vi "PicoReadPicoMultiBuffers.vi"(1 "enabled array":i16[](array[numeric]), 2 "Buffer and Transfer Settings":T3={"startIndex"=0, "Samples"=1000000, "Down Sample Ratio"=1, "Down-Sample Mode"=2147483648} {"Down-Sample Mode" items=["RAW none"=2147483648, "None"=0, "Aggregate"=1, "Decimate"=2, "Average"=4]; "Down Sample Ratio" step=1; "Samples" format="%_6p"}, 3 "Variant":string, 5 "Data Pointers":T1, 9 "No of Buffers":i32=1, 11 "error in (no error)":errorcluster) -> (6 "MultiBuffers (Max or non-aggregated)":T2(array[cluster]), 8 "Min Buffers":T2(array[cluster]), 15 "error out":errorcluster)   [LabVIEW 2024]
doc: "Read data from Picodata buffers for Block and 6000a streaming examples"
uses:
  Buffer and Transfer Settings.ctl
  PicoBuffers.ctl
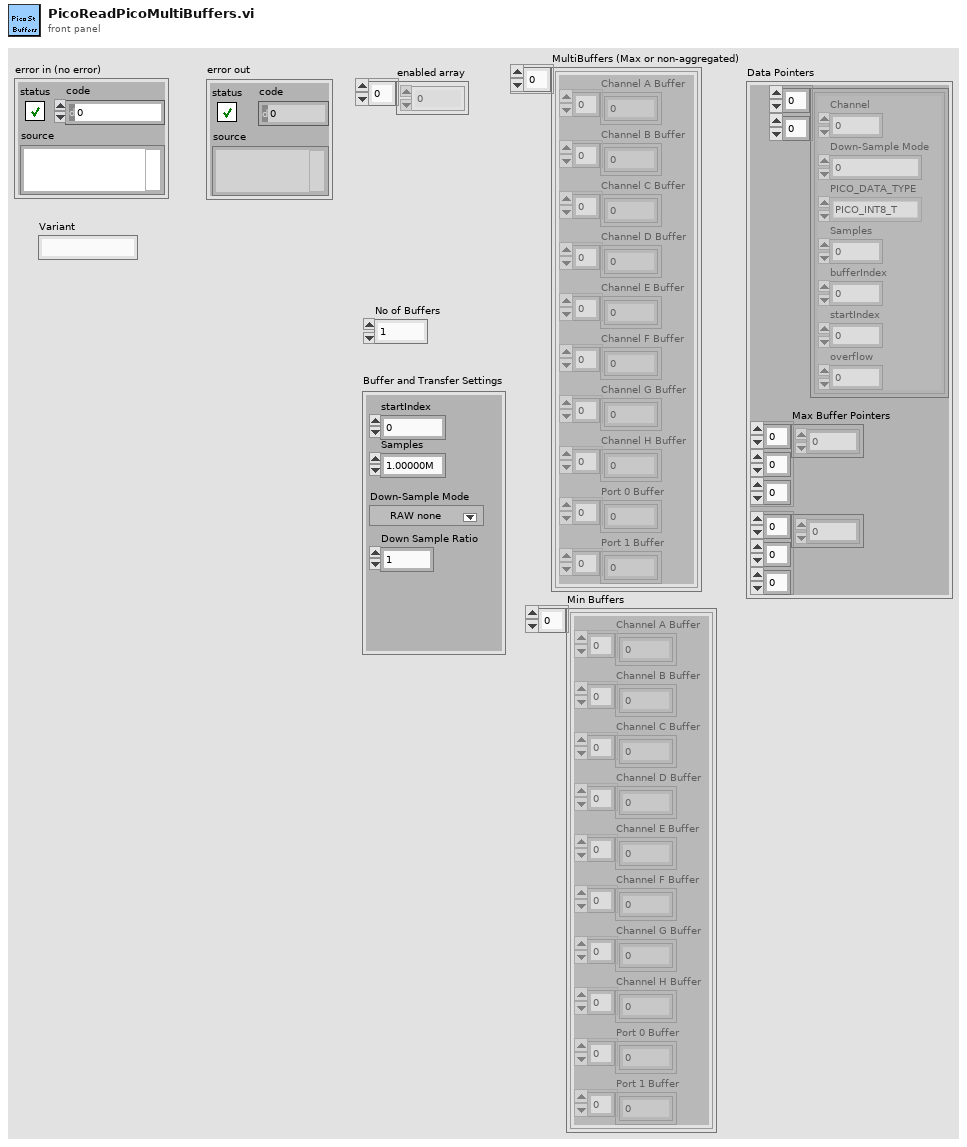
[diagram p1: front panel]
types:
  T1 = typedef "PicoBuffers.ctl" = cluster{"Max Buffer Pointers":u64[][][], "Min Buffer Pointers":u64[][][], "StreamingDataInfo":cluster{"Channel":u32, "Down-Sample Mode":u32, "PICO_DATA_TYPE":enum32{"PICO_INT8_T", "PICO_INT16_T", "PICO_INT32_T", "PICO_UINT32_T", "PICO_INT64_T", ""}, "Samples":i32, "bufferIndex":u64, "startIndex":i32, "overflow":i16}[][]}
  T2 = cluster{"Channel A Buffer":i16[], "Channel B Buffer":i16[], "Channel C Buffer":i16[], "Channel D Buffer":i16[], "Channel E Buffer":i16[], "Channel F Buffer":i16[], "Channel G Buffer":i16[], "Channel H Buffer":i16[], "Port 0 Buffer":i16[], "Port 1 Buffer":i16[]}[]
  T3 = typedef "Buffer and Transfer Settings.ctl" = cluster{"startIndex":u64, "Samples":u64, "Down Sample Ratio":u64, "Down-Sample Mode":u32}
  T4 = cluster{"Channel A Buffer":i16[], "Channel B Buffer":i16[], "Channel C Buffer":i16[], "Channel D Buffer":i16[], "Channel E Buffer":i16[], "Channel F Buffer":i16[], "Channel G Buffer":i16[], "Channel H Buffer":i16[], "Port 0 Buffer":i16[], "Port 1 Buffer":i16[]}
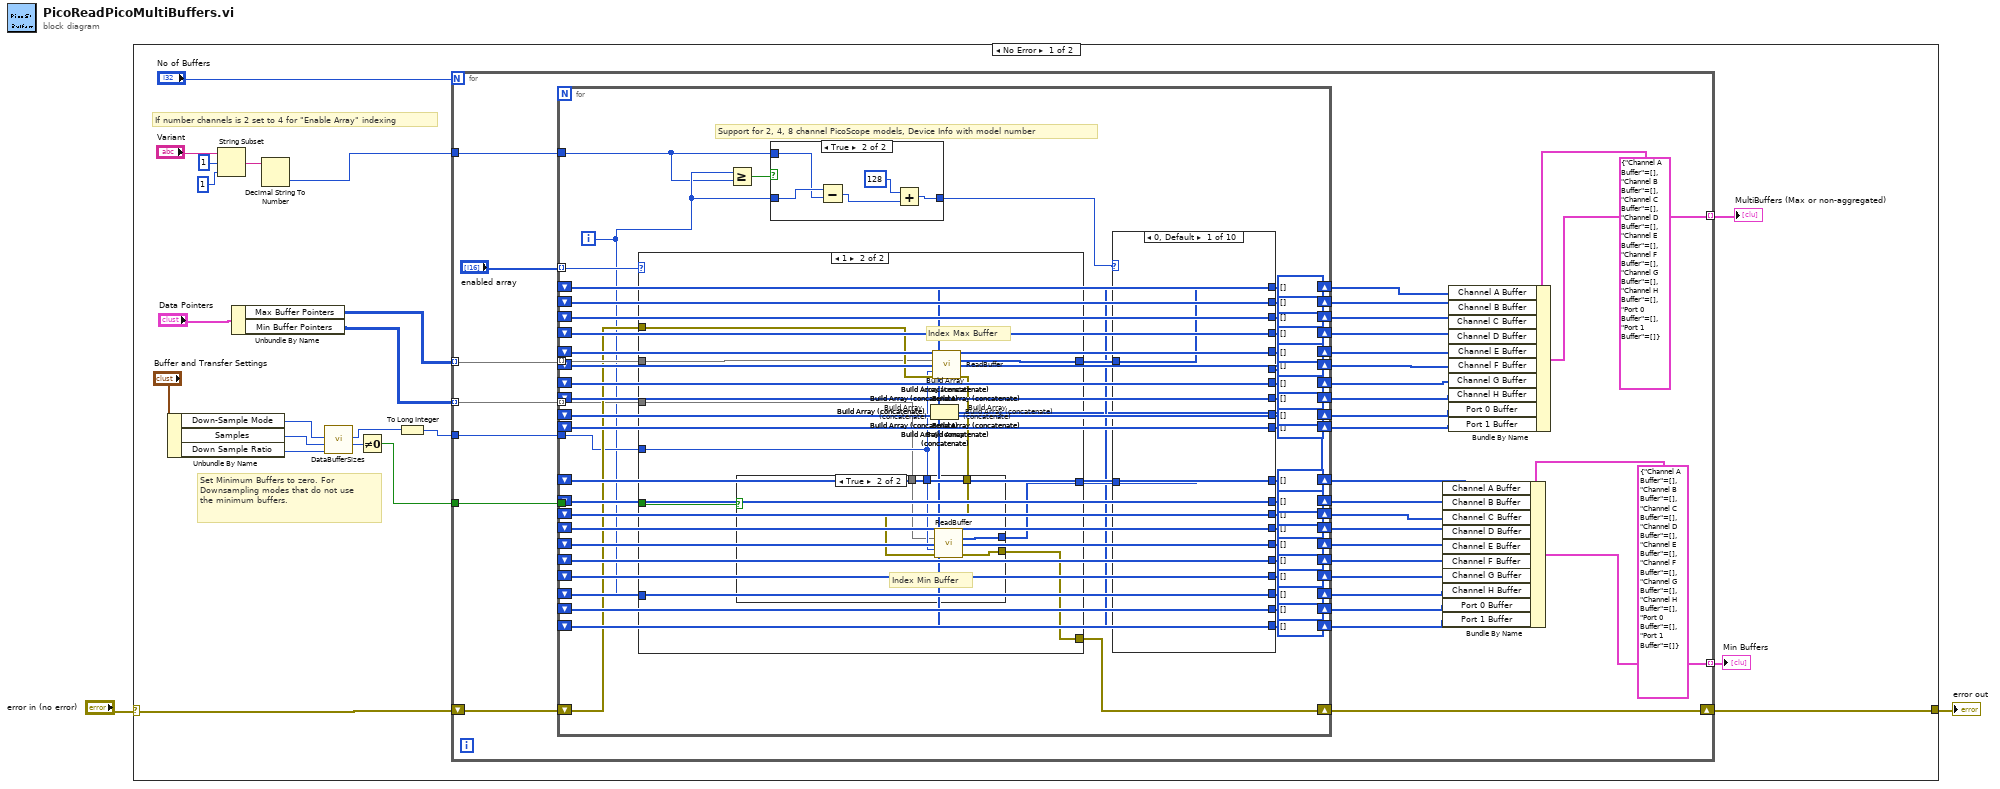
[diagram p0: block diagram]
diagram:
  n1 = case shown="No Error" "error in (no error)" {
    selector: "error in (no error)" -> [w21 w191]
    tunnel: [w23 w191] -> w1
    frame No Error {
      # "If number channels is 2 set to 4 for \"Enable Array\" indexing"
      # "Set Minimum Buffers to zero. For Downsampling modes that do not use the minimum buffers."
      n2 = Unbundle By Name("Buffer and Transfer Settings") -> ("Down-Sample Mode"=w19:u32, "Samples"=w18:u64, "Down Sample Ratio"=w20:u64)
      n3 = String Subset(string="Variant", offset (0)=1, length (rest)=1 ("length (rest)")) -> (substring=w7:string)
      n4 = Unbundle By Name("Data Pointers") -> ("Max Buffer Pointers"=w9:u64[][][], "Min Buffer Pointers"=w8:u64[][][])
      n5 = Decimal String To Number(string=w7) -> (number=w3:i32)  [unwired: 2 in, 1 out]
      n6 = call "DataBufferSizes.vi"("Down Sample Ratio"=w20, "Number of Samples"=w18, "Down-Sample Mode"=w19) -> ("min Buffer Size"=w16:i32, "Max Buffer Size"=w12:i32)  [unwired: 7 in]
      n7 = Not Equal To 0?(x=w16) -> (x != 0?=w17:bool)
      n8 = To Long Integer(number=w12) -> (32bit integer=w15:i32)
      n9 = for {
        N: "No of Buffers" -> [_]
        tunnel: [w73] -> w11 mode=indexing
        tunnel: [w72] -> w13 mode=indexing
        tunnel: w17 -> [w60]
        tunnel: w15 -> [w58]
        shift-right: [w75] -> w23
        shift-left: w21 -> [w74]
        tunnel: w9 -> [w57] mode=indexing
        tunnel: w8 -> [w46] mode=indexing
        tunnel: w3 -> [w45]
        n10 = for {
          tunnel: "enabled array" -> [w147] mode=indexing
          tunnel: w57 -> [w148] mode=indexing
          shift-right: [w146] -> w75
          shift-left: w74 -> [w145]
          tunnel: w58 -> [w131]
          tunnel: w60 -> [w130]
          tunnel: w46 -> [w120] mode=indexing
          tunnel: w45 -> [w116]
          shift-right: [w114] -> w71
          shift-left: i16[] [] ("Output Array") -> [w115]
          shift-right: [w112] -> w70
          shift-left: i16[] [] ("Output Array") -> [w113]
          shift-right: [w110] -> w69
          shift-left: i16[] [] ("Output Array") -> [w111]
          shift-right: [w108] -> w68
          shift-left: i16[] [] ("Output Array") -> [w109]
          shift-right: [w106] -> w67
          shift-left: i16[] [] ("Output Array") -> [w107]
          shift-right: [w104] -> w66
          shift-left: i16[] [] ("Output Array") -> [w105]
          shift-right: [w102] -> w59
          shift-left: i16[] [] ("Output Array") -> [w103]
          shift-right: [w100] -> w65
          shift-left: i16[] [] ("Output Array") -> [w101]
          shift-right: [w98] -> w64
          shift-left: i16[] [] ("Output Array") -> [w99]
          shift-right: [w96] -> w63
          shift-left: i16[] [] ("Output Array") -> [w97]
          shift-right: [w94] -> w62
          shift-left: i16[] [] ("Output Array") -> [w95]
          shift-right: [w92] -> w61
          shift-left: i16[] [] ("Output Array") -> [w93]
          shift-right: [w90] -> w54
          shift-left: i16[] [] ("Output Array") -> [w91]
          shift-right: [w88] -> w53
          shift-left: i16[] [] ("Output Array") -> [w89]
          shift-right: [w86] -> w52
          shift-left: i16[] [] ("Output Array") -> [w87]
          shift-right: [w84] -> w51
          shift-left: i16[] [] ("Output Array") -> [w85]
          shift-right: [w82] -> w50
          shift-left: i16[] [] ("Output Array") -> [w83]
          shift-right: [w80] -> w49
          shift-left: i16[] [] ("Output Array") -> [w81]
          shift-right: [w78] -> w48
          shift-left: i16[] [] ("Output Array") -> [w79]
          shift-right: [w76] -> w47
          shift-left: i16[] [] ("Output Array") -> [w77]
          i -> [w117]
          # "Support for 2, 4, 8 channel PicoScope models, Device Info with model number"
          n11 = case shown="1" w147 {
            tunnel: w148 -> [_ w177]
            tunnel: w117 -> [_ _]
            tunnel: [_ w184] -> w144
            tunnel: [_ w183] -> w143
            tunnel: w145 -> [w175 w182]
            tunnel: [w175 w180] -> w146
            tunnel: w131 -> [_ w178]
            tunnel: w130 -> [_ w179]
            tunnel: w120 -> [_ w176]
            frame 0, Default {
            }
            frame 1 {
              # "Index Max Buffer"
              n12 = call "ReadBuffer.vi"("Pointer and BufferSize"=w177, "Buffer size"=w178, "error in (no error)"=w182) -> ("Output Array"=w184:i16[], "error out"=w181:errorcluster)  [unwired: 11 in]
              n13 = case shown="True" w179 {
                tunnel: [_ w190] -> w183
                tunnel: w181 -> [w185 w189]
                tunnel: [w185 w188] -> w180
                tunnel: w178 -> [_ w187]
                tunnel: w176 -> [_ w186]
                frame False {
                }
                frame True {
                  # "Index Min Buffer"
                  n14 = call "ReadBuffer.vi"("Pointer and BufferSize"=w186, "Buffer size"=w187, "error in (no error)"=w189) -> ("Output Array"=w190:i16[], "error out"=w188:errorcluster)  [unwired: 11 in]
                }
              }
            }
          }
          n15 = Greater Or Equal?(x=w117, y=w116) -> (x >= y?=w119:bool)
          n16 = case shown="True" w119 {
            tunnel: w117 -> [w149 w151]
            tunnel: [w149 w153] -> w118
            tunnel: w116 -> [_ w150]
            frame False {
            }
            frame True {
              n17 = Subtract(x=w151, y=w150) -> (x-y=w152:i32)
              n18 = Add(x=128, y=w152) -> (x+y=w153:i32)
            }
          }
          n19 = case shown="0, Default" w118 {
            tunnel: w144 -> [w156 w158 w160 w162 w164 w166 w168 w170 w172 w174]
            tunnel: [w156 _ _ _ _ _ _ _ _ _] -> w129
            tunnel: [_ w158 _ _ _ _ _ _ _ _] -> w136
            tunnel: [_ _ w160 _ _ _ _ _ _ _] -> w135
            tunnel: [_ _ _ w162 _ _ _ _ _ _] -> w134
            tunnel: [_ _ _ _ w164 _ _ _ _ _] -> w133
            tunnel: [_ _ _ _ _ w166 _ _ _ _] -> w132
            tunnel: w143 -> [w155 w157 w159 w161 w163 w165 w167 w169 w171 w173]
            tunnel: [w155 _ _ _ _ _ _ _ _ _] -> w142
            tunnel: [_ w157 _ _ _ _ _ _ _ _] -> w141
            tunnel: [_ _ w159 _ _ _ _ _ _ _] -> w140
            tunnel: [_ _ _ w161 _ _ _ _ _ _] -> w139
            tunnel: [_ _ _ _ w163 _ _ _ _ _] -> w138
            tunnel: [_ _ _ _ _ w165 _ _ _ _] -> w137
            tunnel: [_ _ _ _ _ _ w168 _ _ _] -> w128
            tunnel: [_ _ _ _ _ _ w167 _ _ _] -> w127
            tunnel: [_ _ _ _ _ _ _ w170 _ _] -> w126
            tunnel: [_ _ _ _ _ _ _ w169 _ _] -> w125
            tunnel: [_ _ _ _ _ _ _ _ w172 _] -> w124
            tunnel: [_ _ _ _ _ _ _ _ w171 _] -> w123
            tunnel: [_ _ _ _ _ _ _ _ _ w174] -> w122
            tunnel: [_ _ _ _ _ _ _ _ _ w173] -> w121
            frame 0, Default {
            }
            frame 1 {
            }
            frame 2 {
            }
            frame 3 {
            }
            frame 4 {
            }
            frame 5 {
            }
            frame 6 {
            }
            frame 7 {
            }
            frame 128 {
            }
            frame 129 {
            }
          }
          n20 = Build Array (concatenate)(w77, w121) -> (w76:i16[])
          n21 = Build Array (concatenate)(w79, w122) -> (w78:i16[])
          n22 = Build Array (concatenate)(w81, w123) -> (w80:i16[])
          n23 = Build Array (concatenate)(w83, w124) -> (w82:i16[])
          n24 = Build Array (concatenate)(w85, w125) -> (w84:i16[])
          n25 = Build Array (concatenate)(w87, w126) -> (w86:i16[])
          n26 = Build Array (concatenate)(w89, w127) -> (w88:i16[])
          n27 = Build Array (concatenate)(w91, w128) -> (w90:i16[])
          n28 = Build Array (concatenate)(w93, w132) -> (w92:i16[])
          n29 = Build Array (concatenate)(w95, w133) -> (w94:i16[])
          n30 = Build Array (concatenate)(w97, w134) -> (w96:i16[])
          n31 = Build Array (concatenate)(w99, w135) -> (w98:i16[])
          n32 = Build Array (concatenate)(w101, w136) -> (w100:i16[])
          n33 = Build Array (concatenate)(w103, w129) -> (w102:i16[])
          n34 = Build Array (concatenate)(w105, w137) -> (w104:i16[])
          n35 = Build Array (concatenate)(w107, w138) -> (w106:i16[])
          n36 = Build Array (concatenate)(w109, w139) -> (w108:i16[])
          n37 = Build Array (concatenate)(w111, w140) -> (w110:i16[])
          n38 = Build Array (concatenate)(w113, w141) -> (w112:i16[])
          n39 = Build Array (concatenate)(w115, w142) -> (w114:i16[])
        }
        n40 = Bundle By Name(cluster=T4 {"Channel A Buffer"=[], "Channel B Buffer"=[], "Channel C Buffer"=[], "Channel D Buffer"=[], "Channel E Buffer"=[], "Channel F Buffer"=[], "Channel G Buffer"=[], "Channel H Buffer"=[], "Port 0 Buffer"=[], "Port 1 Buffer"=[]} ("input cluster"), "Channel A Buffer"=w71, "Channel B Buffer"=w70, "Channel C Buffer"=w69, "Channel D Buffer"=w68, "Channel E Buffer"=w67, "Channel F Buffer"=w66, "Channel G Buffer"=w53, "Channel H Buffer"=w51, "Port 0 Buffer"=w49, "Port 1 Buffer"=w47) -> (w73:T4)
        n41 = Bundle By Name(cluster=T4 {"Channel A Buffer"=[], "Channel B Buffer"=[], "Channel C Buffer"=[], "Channel D Buffer"=[], "Channel E Buffer"=[], "Channel F Buffer"=[], "Channel G Buffer"=[], "Channel H Buffer"=[], "Port 0 Buffer"=[], "Port 1 Buffer"=[]} ("input cluster"), "Channel A Buffer"=w59, "Channel B Buffer"=w65, "Channel C Buffer"=w64, "Channel D Buffer"=w63, "Channel E Buffer"=w62, "Channel F Buffer"=w61, "Channel G Buffer"=w54, "Channel H Buffer"=w52, "Port 0 Buffer"=w50, "Port 1 Buffer"=w48) -> (w72:T4)
      }
      "MultiBuffers (Max or non-aggregated)" <- w13
      "Min Buffers" <- w11
    }
    frame Error {
    }
  }
  "error out" <- w1
